vi "Test.vi"(10 "Class Select":enum16{"DMM", "Power_Supply"}(ring), 11 "User Reference":T1) -> (0 "error out":errorcluster, 3 "Class Attributes":T2)   [LabVIEW 2018]
uses:
  Controls/Class Attributes Cluster.ctl
  Controls/User Reference.ctl
  Power_Supply/Power_Supply Virtual/Power_Supply Virtual.lvclass
  DMM/DMM Virtual/DMM Virtual.lvclass
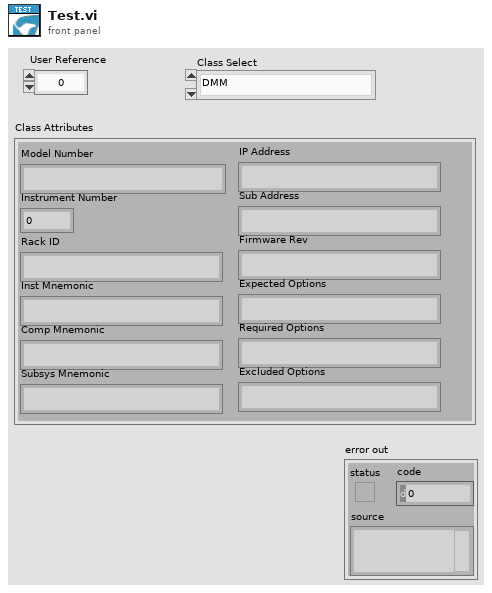
[diagram p1: front panel]
types:
  T1 = typedef "User Reference.ctl" = i32
  T2 = typedef "Class Attributes Cluster.ctl" = cluster{"Model Number":string, "Instrument Number":u8, "Rack ID":string, "Inst Mnemonic":string, "Comp Mnemonic":string, "Subsys Mnemonic":string, "IP Address":string, "Sub Address":string, "Firmware Rev":string, "Expected Options":string, "Required Options":string, "Excluded Options":string}
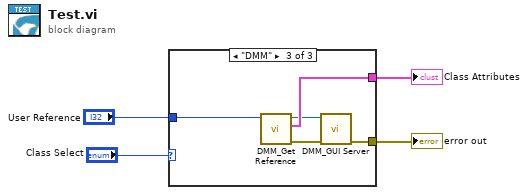
[diagram p0: block diagram]
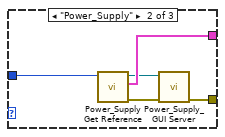
[diagram p3: hidden frame]
diagram:
  n1 = case shown="\"DMM\"" "Class Select" {
    tunnel: "User Reference" -> [_ w9 w14]
    tunnel: [_ w5 w10] -> w4
    tunnel: [_ w8 w13] -> w3
    frame Default {
    }
    frame "Power_Supply" {
      n2 = call "Power_Supply Get Reference.vi"("Instrument Reference"=w9) -> ("error out"=w6:errorcluster, "Class Attributes"=w8:T2, "Power_Supply Virtual.lvclass"=w7:refnum<class "Power_Supply Virtual.lvclass">)  [unwired: 8 in]
      n3 = call-dynamic "Power_Supply_GUI Server.vi"("error in (no error)"=w6, "Power_Supply Virtual in"=w7) -> ("error out"=w5:errorcluster)  [unwired: 8 in, 1 out]
    }
    frame "DMM" {
      n4 = call "DMM_Get Reference.vi"("Instrument Reference"=w14) -> ("error out"=w11:errorcluster, "Class Attributes"=w13:T2, "DMM Virtual.lvclass"=w12:refnum<class "DMM Virtual.lvclass">)  [unwired: 8 in]
      n5 = call-dynamic "DMM_GUI Server.vi"("error in (no error)"=w11, "DMM Virtual in"=w12) -> ("error out"=w10:errorcluster)  [unwired: 8 in, 1 out]
    }
  }
  "error out" <- w4
  "Class Attributes" <- w3
